vi "subDFD_Set Busy VI.vi"(8 "error in (no error)":errorcluster, 10 "busy task":string, 11 "Busy vi reference":refnum<vi>) -> (0 "error out":errorcluster, 3 "dup Busy vi reference":refnum<vi>)   [LabVIEW 2017]
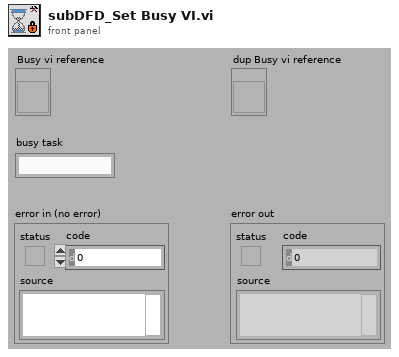
[diagram p1: front panel]
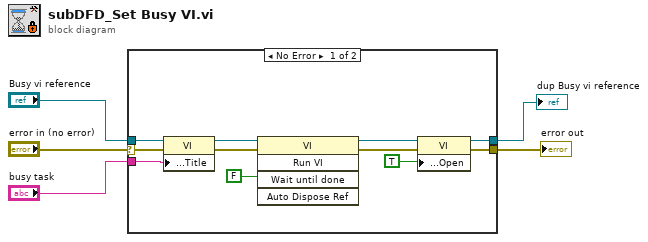
[diagram p0: block diagram]
diagram:
  n1 = case shown="No Error" "error in (no error)" {
    selector: "error in (no error)" -> [w6 w18]
    tunnel: [w12 w17] -> w5
    tunnel: [w11 w18] -> w4
    tunnel: "Busy vi reference" -> [w10 w17]
    tunnel: "busy task" -> [w7 _]
    frame No Error {
      n2 = property class="VI"(reference=w10, error in=w6, "Front Panel.Title"=w7) -> (reference out=w9:refnum<vi>, error out=w8:errorcluster)
      n3 = invoke class="VI" method="Run VI"(reference=w9, error in=w8, "Wait until done"=FALSE ("Wait Until Done")) -> (reference out=w15:refnum<vi>, error out=w14:errorcluster)  [unwired: 2 in, 3 out]
      n4 = property class="VI"(reference=w15, error in=w14, "Front Panel.Open"=TRUE ("Front Panel Window:Open")) -> (reference out=w12:refnum<vi>, error out=w11:errorcluster)
    }
    frame Error {
    }
  }
  "dup Busy vi reference" <- w5
  "error out" <- w4
